vi "lower version vi.vi"(8 "Numeric":dbl=25.0) -> (0 "x+y":dbl)   [LabVIEW 2016]
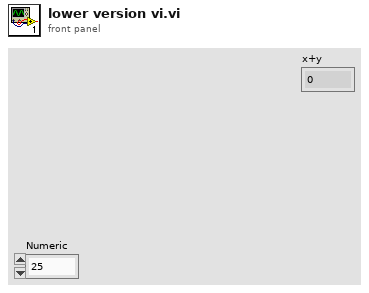
[diagram p1: front panel]
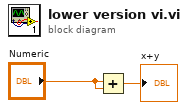
[diagram p0: block diagram]
diagram:
  n1 = Add(x="Numeric", y="Numeric") -> (x+y=→"x+y":dbl)
